vi "Temp_konwersja.vi"(8 "error in (no error)":errorcluster, 10 "Temp in":dbl) -> (0 "error out":errorcluster, 2 "Temp out":dbl)   [LabVIEW 2013]
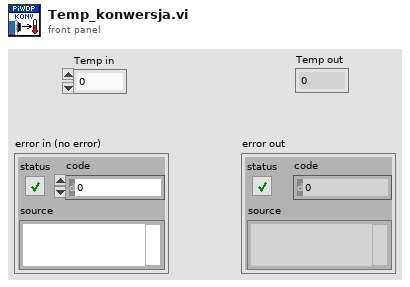
[diagram p1: front panel]
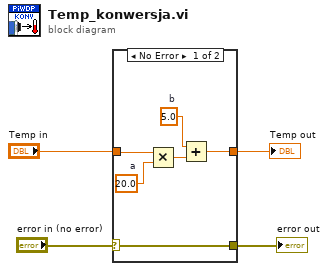
[diagram p0: block diagram]
diagram:
  n1 = case shown="No Error" "error in (no error)" {
    selector: "error in (no error)" -> [w10 w11]
    tunnel: "Temp in" -> [w9 w12]
    tunnel: [w10 w11] -> w2
    tunnel: [w7 w12] -> w1
    frame No Error {
      w5 = 5.0  # b
      w6 = 20.0  # a
      n2 = Multiply(x=w9, y=w6) -> (x*y=w8:dbl)
      n3 = Add(x=w5, y=w8) -> (x+y=w7:dbl)
    }
    frame Error {
    }
  }
  "Temp out" <- w1
  "error out" <- w2
